vi "Charge Injection Limit Calculation.vi"(8 "appended array":dbl[](array[numeric]), 9 "Em(phase2)":dbl[](array[numeric]), 10 "Em(phase 1)":dbl[](array[numeric]), 11 "Measurements":dbl[](array[numeric])) -> (0 "Em(phase2) Ind":dbl[](array[numeric]), 1 "CIL":cluster{"appended array":dbl[], dbl[]}[](array[cluster]), 2 "Em(phase 1) ind":dbl[](array[numeric]), 3 "appended array ind":dbl[](array[numeric]))   [LabVIEW 2022 SP3]
panel:
  in  "Measurements 2":dbl[](array[numeric])
  in  "Inter-phase Duration (us)":u32=50
  in  "Duration (us) Phase 1":u32=300
  in  "Pre Stim Recording Duration (us)":u32=50
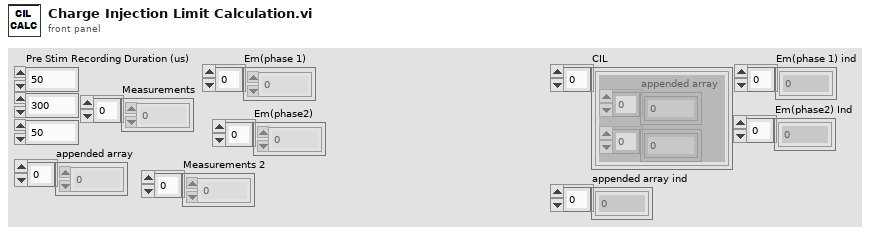
[diagram p1: front panel]
types:
  T1 = cluster{"appended array":dbl[], "appended array":dbl[]}[]
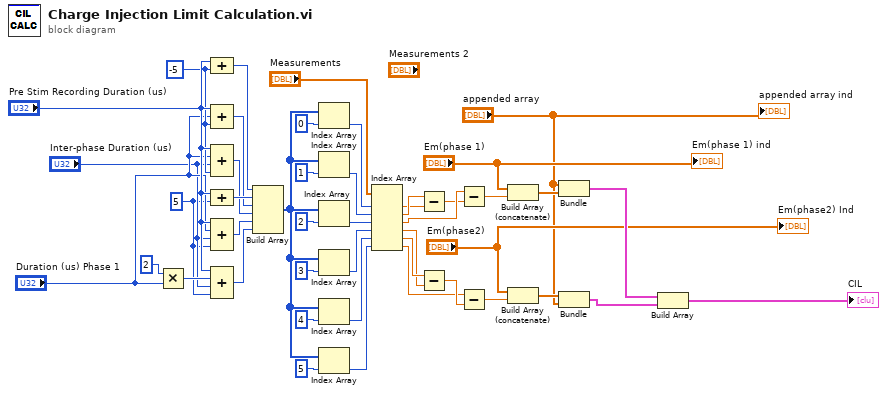
[diagram p0: block diagram]
diagram:
  w32 = -5
  w27 = 5
  n1 = Multiply(x=2, y="Duration (us) Phase 1") -> (x*y=w29:u32)
  n2 = Compound Arithmetic op=ADD("Pre Stim Recording Duration (us)", w32) -> (w26:u32)
  n3 = Compound Arithmetic op=ADD("Pre Stim Recording Duration (us)", "Duration (us) Phase 1", w32) -> (w24:u32)
  n4 = Compound Arithmetic op=ADD("Pre Stim Recording Duration (us)", "Duration (us) Phase 1", "Inter-phase Duration (us)", w32) -> (w23:u32)
  n5 = Compound Arithmetic op=ADD("Pre Stim Recording Duration (us)", w27) -> (w25:u32)
  n6 = Compound Arithmetic op=ADD("Pre Stim Recording Duration (us)", "Duration (us) Phase 1", "Inter-phase Duration (us)", w27) -> (w22:u32)
  n7 = Compound Arithmetic op=ADD("Pre Stim Recording Duration (us)", w29, "Inter-phase Duration (us)", w27) -> (w21:u32)
  n8 = Build Array(w26, w25, w24, w23, w22, w21) -> (w20:u32[])
  n9 = Index Array(array=w20, index=0) -> (element=w34:u32)
  n10 = Index Array(array=w20, index=1) -> (element=w35:u32)
  n11 = Index Array(array=w20, index=2) -> (element=w36:u32)
  n12 = Index Array(array=w20, index=3) -> (element=w37:u32)
  n13 = Index Array(array=w20, index=4) -> (element=w38:u32)
  n14 = Index Array(array=w20, index=5) -> (element=w39:u32)
  n15 = Index Array(array="Measurements", index #1=w34, index #2=w35, index #3=w36, index #4=w37, index #5=w38, index #6=w39) -> (element #1=w18:dbl, element #2=w19:dbl, element #3=w14:dbl, element #4=w15:dbl, element #5=w16:dbl, element #6=w11:dbl)
  n16 = Subtract(x=w19, y=w18) -> (x-y=w13:dbl)
  n17 = Subtract(x=w16, y=w15) -> (x-y=w12:dbl)
  n18 = Subtract(x=w14, y=w13) -> (x-y=w10:dbl)
  n19 = Subtract(x=w11, y=w12) -> (x-y=w6:dbl)
  n20 = Build Array (concatenate)("Em(phase 1)", w10) -> (w5:dbl[])
  n21 = Build Array (concatenate)("Em(phase2)", w6) -> (w4:dbl[])
  n22 = Bundle("appended array"="appended array", w5) -> (w9:cluster{"appended array":dbl[], dbl[]})  [unwired: 1 in]
  n23 = Bundle(w4, "appended array"="appended array") -> (w1:cluster{dbl[], "appended array":dbl[]})  [unwired: 1 in]
  n24 = Build Array(w9, w1) -> (→"CIL":T1)
  "appended array ind" <- "appended array"
  "Em(phase 1) ind" <- "Em(phase 1)"
  "Em(phase2) Ind" <- "Em(phase2)"
